vi "Initialize.vi"(8 "Error In":errorcluster) -> (0 "Error Out":errorcluster)   [LabVIEW 2018, in "StopUE.lvlib"]
uses:
  StopUE.lvlib
  States_FGV.ctl
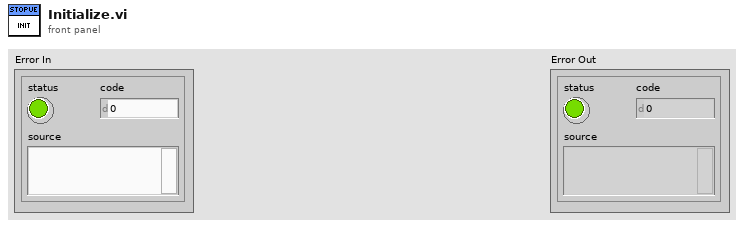
[diagram p1: front panel]
types:
  T1 = typedef "StopUE.lvlib/States_FGV.ctl" = enum16{"Get", "Shutdown", "Initialize"}
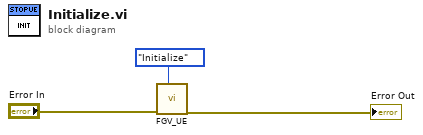
[diagram p0: block diagram]
diagram:
  n1 = call "FGV_UE.vi"("State"=States_FGV."Initialize", "Error In"="Error In") -> ("Error Out"=→"Error Out":errorcluster)  [unwired: 8 in, 1 out]
